vi "AP Quiz From File.vi"(8 "Error In":errorcluster, 11 "file path (dialog if empty)":path=path "C:/Users/husmith/Documents/GitHub/Action Pack/Quiz/QuizSetupSpreadsheet_Test.txt") -> (0 "Error Out":errorcluster, 1 "Raw Data":string[][](array[string]), 2 "Question Array Out":T1[](array[typedef]))   [LabVIEW 2012]
uses:
  Controls/Quiz Info.ctl
  Controls/Quiz Solution.ctl
  <vilib>/Utility/file.llb/Read From Spreadsheet File (string).vi
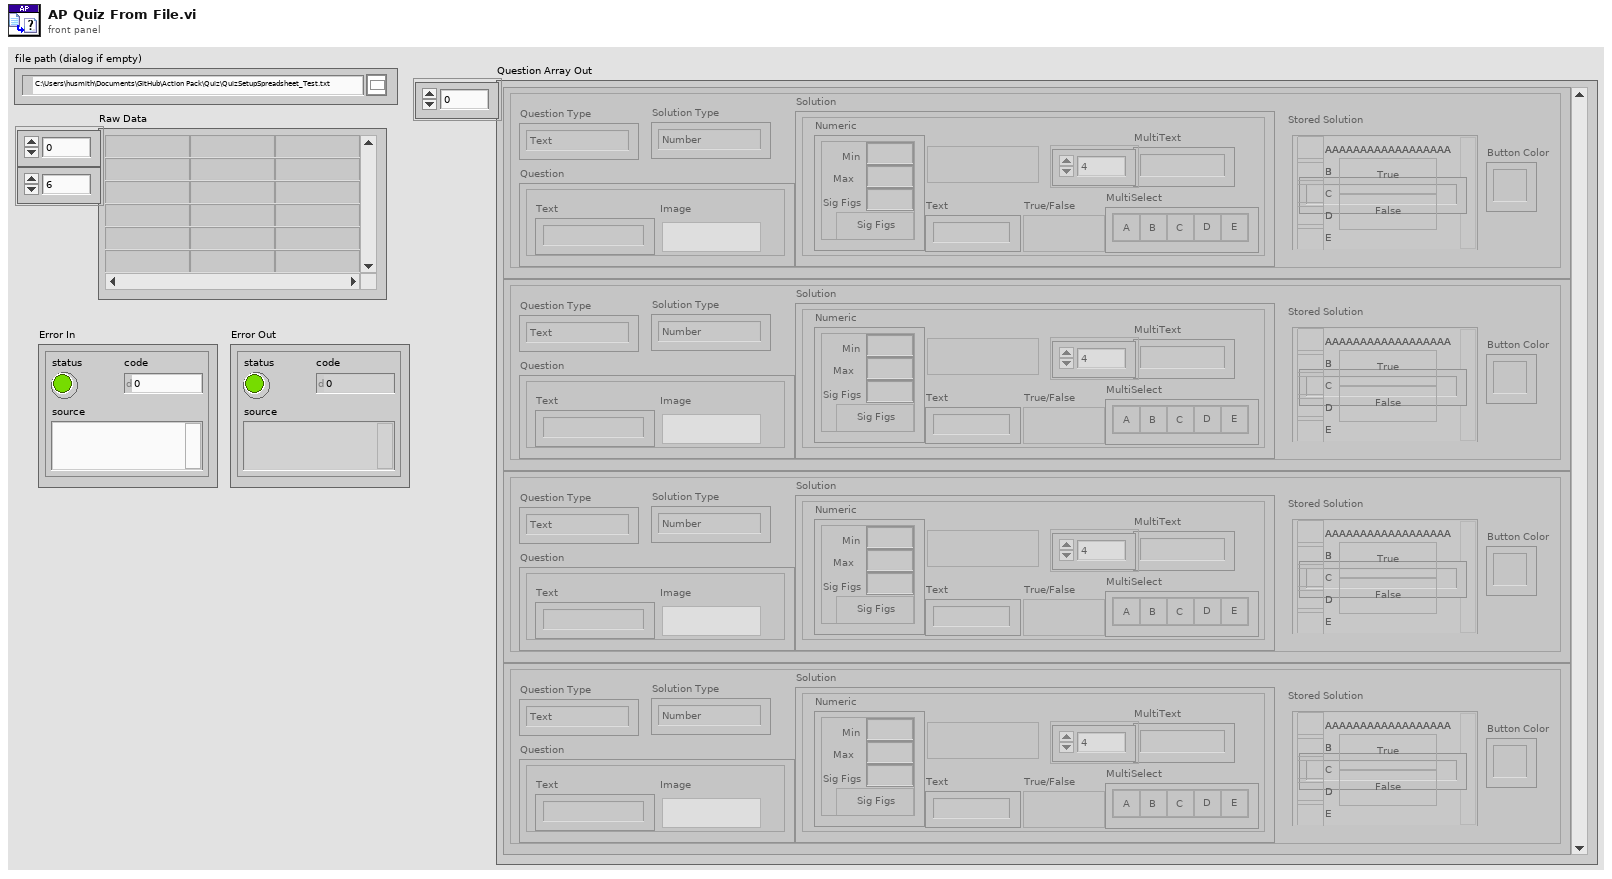
[diagram p1: front panel]
types:
  T1 = typedef "Quiz Info.ctl" = cluster{"Question Type":enum16{"Text", "Image", "Text&Image"}, "Solution Type":enum16{"Number", "Text", "MultiChoice", "Radio", "T/F", "Paragraph"}, "Question":cluster{"Text":string, "Image":picture}, "Solution":cluster{"Numeric":cluster{"Min":dbl, "Max":dbl, "Sig Figs":i32, "Sig Figs?":bool}, "Text":string, "True/False":bool, "MultiSelect":cluster{"A":bool, "B":bool, "C":bool, "D":bool, "E":bool}, "MultiText":string[], "Text Case Match":bool}, "Stored Solution":T2, "Button Color":u32}
  T2 = typedef "Quiz Solution.ctl" = cluster{"Numeric":dbl, "Text":string, "Multi":cluster{"A":bool, "B":bool, "C":bool, "D":bool, "E":bool}, "Radio":enum32{"No Selection", "A", "B", "C", "D", "E"}, "True/False":enum32{"No Selection", "True", "False"}, "Short Answer":string}
  T3 = enum16{"Number", "Text", "MultiChoice", "Radio", "T/F", "Paragraph"}
  T4 = typedef "imagedata.ctl" = cluster{"image type":i32, "image depth":i32, "image":u8[], "mask":u8[], "colors":u32[], "Rectangle":cluster{"left":i16, "top":i16, "right":i16, "bottom":i16}}
  T5 = cluster{"A":bool, "B":bool, "C":bool, "D":bool, "E":bool}
  T6 = cluster{"MultiSelect[0]":bool, "MultiSelect[1]":bool, "MultiSelect[2]":bool, "MultiSelect[3]":bool, "MultiSelect[4]":bool}
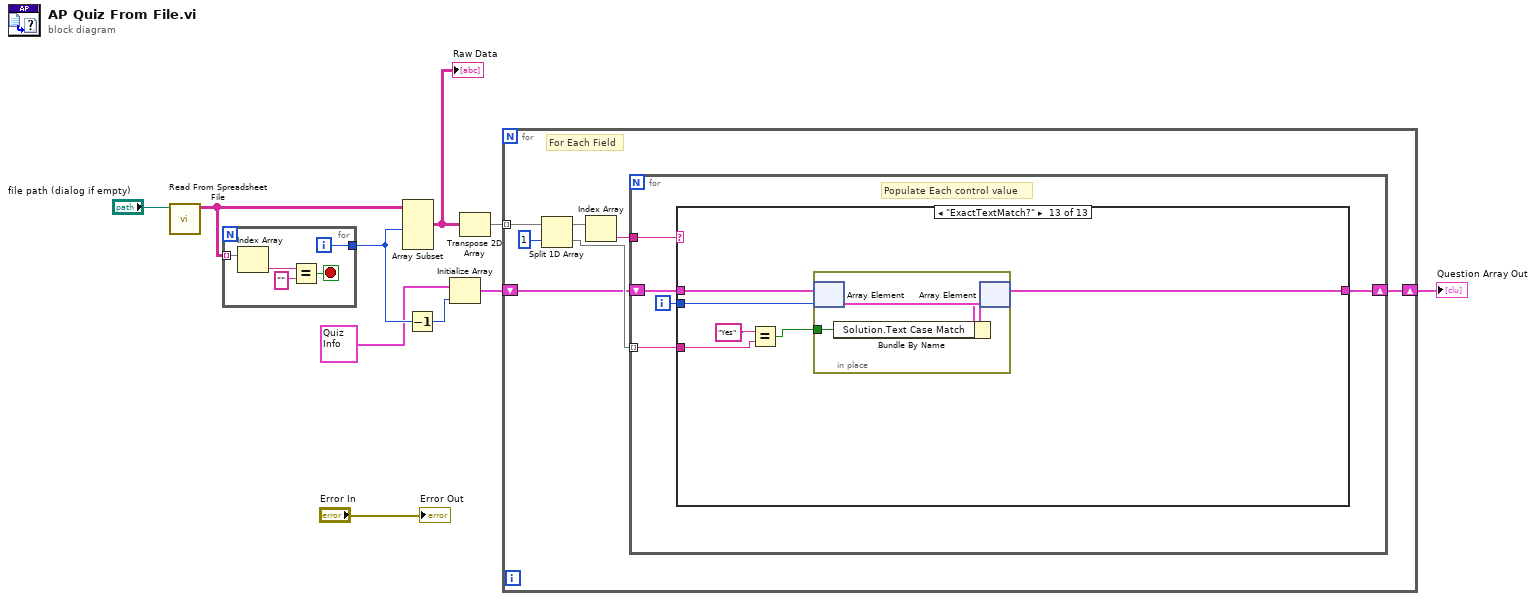
[diagram p0: block diagram]
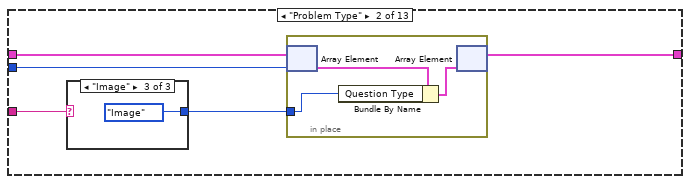
[diagram p3: hidden frame]
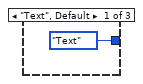
[diagram p4: hidden frame]
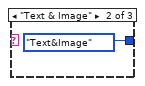
[diagram p5: hidden frame]
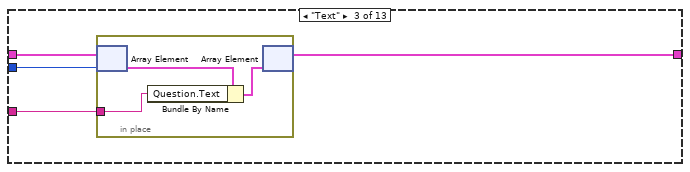
[diagram p6: hidden frame]
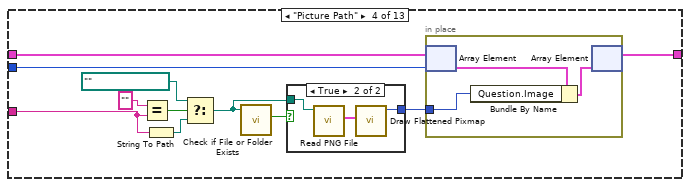
[diagram p7: hidden frame]
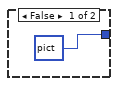
[diagram p8: hidden frame]
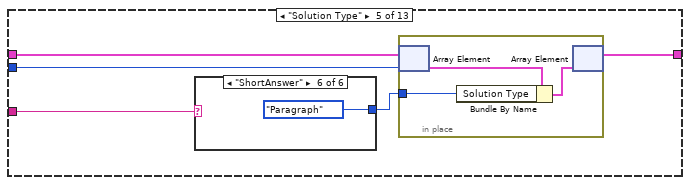
[diagram p9: hidden frame]
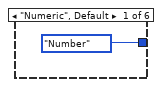
[diagram p10: hidden frame]
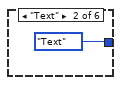
[diagram p11: hidden frame]
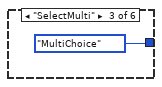
[diagram p12: hidden frame]
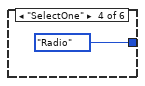
[diagram p13: hidden frame]
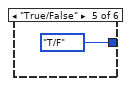
[diagram p14: hidden frame]
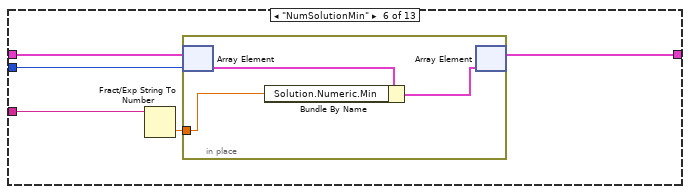
[diagram p15: hidden frame]
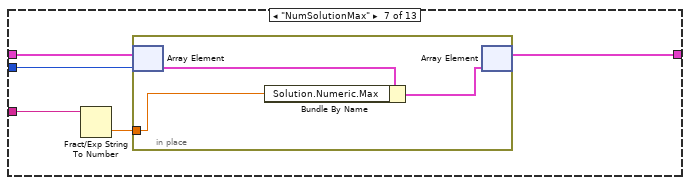
[diagram p16: hidden frame]
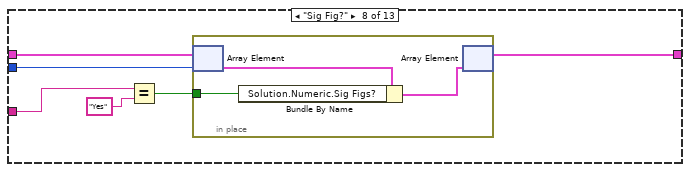
[diagram p17: hidden frame]
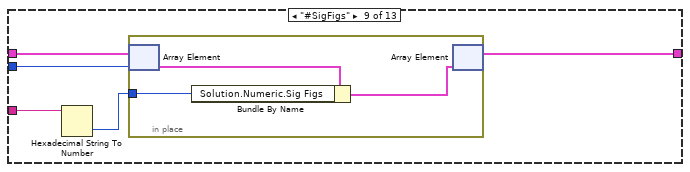
[diagram p18: hidden frame]
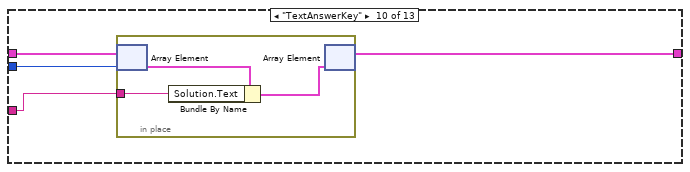
[diagram p19: hidden frame]
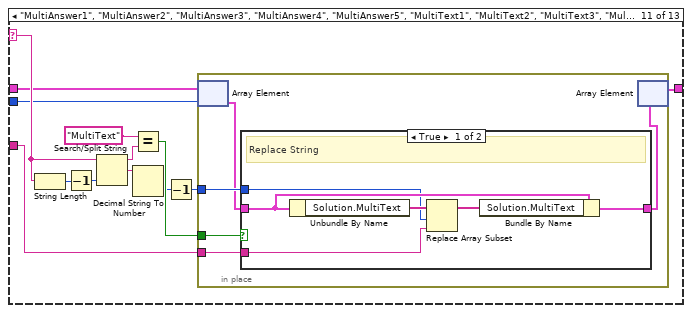
[diagram p20: hidden frame]
diagram:
  n1 = call-poly <vilib>:"Read From Spreadsheet File.vi"("file path (dialog if empty)"="file path (dialog if empty)") -> ("all rows"=w9:string[][])  [unwired: 6 in, 4 out]
  n2 = for {
    tunnel: [w14] -> w6
    tunnel: w9 -> [w13] mode=indexing
    i -> [w14]
    stop <- w11 stop-if-true
    n3 = Index Array(array=w13) -> (element=w12:string)  [unwired: 1 in]
    n4 = Equal?(x=w12, y="") -> (x = y?=w11:bool)
  }
  n5 = Array Subset(array=w9, length (row)=w6) -> (w5:string[][])  [unwired: 3 in]
  "Raw Data" <- w5
  n6 = Decrement(x=w6) -> (x-1=w7:i32)
  n7 = Initialize Array(T1 {"Question Type"=enum."Text", "Solution Type"=enum."Number", "Question"={"Text"="", "Image"=bytes[0]}, "Solution"={"Numeric"={"Min"=0.0, "Max"=0.0, "Sig Figs"=0, "Sig Figs?"=FALSE}, "Text"="", "True/False"=FALSE, "MultiSelect"={"A"=FALSE, "B"=FALSE, "C"=FALSE, "D"=FALSE, "E"=FALSE}, "MultiText"=["", "", "", "", ""], "Text Case Match"=FALSE}, "Stored Solution"={"Numeric"=0.0, "Text"="", "Multi"={"A"=FALSE, "B"=FALSE, "C"=FALSE, "D"=FALSE, "E"=FALSE}, "Radio"=enum."No Selection", "True/False"=enum."No Selection", "Short Answer"=""}, "Button Color"=14869218} ("Quiz Info"), w7) -> (w8:T1[])
  n8 = Transpose 2D Array(2D array=w5) -> (transposed array=w10:string[][])
  n9 = for {
    tunnel: w10 -> [w22] mode=indexing
    shift-right: [w16] -> w1
    shift-left: w8 -> [w18]
    # "For Each Field"
    n10 = Split 1D Array(array=w22, index=1) -> (first subarray=w19:string[], second subarray=w20:string[])
    n11 = Index Array(array=w19) -> (element=w17:string)  [unwired: 1 in]
    n12 = for {
      tunnel: w20 -> [w27] mode=indexing
      tunnel: w17 -> [w26]
      shift-right: [w24] -> w16
      shift-left: w18 -> [w25]
      i -> [w23]
      # "Populate Each control value"
      n13 = case shown="\"ExactTextMatch?\"" w26 {
        selector: w26 -> [_ _ _ _ _ _ _ _ _ _ w126 _ _]
        tunnel: w27 -> [_ w33 w40 w52 w67 w83 w91 w97 w105 w112 w120 w155 w164]
        tunnel: w25 -> [w28 w32 w43 w56 w69 w81 w89 w99 w107 w114 w125 w157 w167]
        tunnel: [w28 w31 w42 w57 w68 w79 w87 w98 w106 w113 w119 w158 w166] -> w24
        tunnel: w23 -> [_ w29 w41 w54 w65 w82 w90 w100 w108 w115 w124 w156 w162]
        frame "NULL", Default {
        }
        frame "Problem Type" {
          n14 = case shown="\"Image\"" w33 {
            tunnel: [enum16{"Text", "Image", "Text&Image"}."Text" ("Question Type") enum16{"Text", "Image", "Text&Image"}."Text&Image" ("Question Type") enum16{"Text", "Image", "Text&Image"}."Image" ("Question Type")] -> w30
            frame "Text", Default {
            }
            frame "Text & Image" {
            }
            frame "Image" {
            }
          }
          n15 = in-place {
            in-place-border: w30 -> [w34]
            n16 = in-place-array #1(w32, w29) -> (w36:T1)
            n17 = Bundle By Name(cluster=w36, "Question Type"=w34) -> (w35:T1)
            n18 = in-place-array #1(w35) -> (w31:T1[])  [unwired: 1 out]
          }
        }
        frame "Text" {
          n19 = in-place {
            in-place-border: w40 -> [w44]
            n20 = in-place-array #2(w43, w41) -> (w46:T1)
            n21 = Bundle By Name(cluster=w46, "Question.Text"=w44) -> (w45:T1)
            n22 = in-place-array #2(w45) -> (w42:T1[])  [unwired: 1 out]
          }
        }
        frame "Picture Path" {
          n23 = Equal?(x="", y=w52) -> (x = y?=w50:bool)
          n24 = String To Path(string=w52) -> (path=w49:path)
          n25 = Select(t=path "", s=w50, f=w49) -> (s? t:f=w48:path)
          n26 = call <vilib>:"Check if File or Folder Exists.vi"("path"=w48) -> ("file or folder exists?"=w53:bool)  [unwired: 8 in, 2 out]
          n27 = case shown="True" w53 {
            tunnel: [picture data[5B] ("new picture") w60] -> w55
            tunnel: w48 -> [_ w59]
            frame False {
            }
            frame True {
              n28 = call <vilib>:"Read PNG File.vi"("path to PNG file"=w59) -> ("image data"=w61:T4)  [unwired: 8 in, 2 out]
              n29 = call <vilib>:"Draw Flattened Pixmap.vi"("image data"=w61) -> ("new picture"=w60:picture)  [unwired: 8 in]
            }
          }
          n30 = in-place {
            in-place-border: w55 -> [w62]
            n31 = in-place-array #3(w56, w54) -> (w64:T1)
            n32 = Bundle By Name(cluster=w64, "Question.Image"=w62) -> (w63:T1)
            n33 = in-place-array #3(w63) -> (w57:T1[])  [unwired: 1 out]
          }
        }
        frame "Solution Type" {
          n34 = case shown="\"ShortAnswer\"" w67 {
            tunnel: [T3."Number" ("Solution Type") T3."Text" ("Solution Type") T3."MultiChoice" ("Solution Type") T3."Radio" ("Solution Type") T3."T/F" ("Solution Type") T3."Paragraph" ("Solution Type")] -> w66
            frame "Numeric", Default {
            }
            frame "Text" {
            }
            frame "SelectMulti" {
            }
            frame "SelectOne" {
            }
            frame "True/False" {
            }
            frame "ShortAnswer" {
            }
          }
          n35 = in-place {
            in-place-border: w66 -> [w76]
            n36 = in-place-array #4(w69, w65) -> (w78:T1)
            n37 = Bundle By Name(cluster=w78, "Solution Type"=w76) -> (w77:T1)
            n38 = in-place-array #4(w77) -> (w68:T1[])  [unwired: 1 out]
          }
        }
        frame "NumSolutionMin" {
          n39 = Fract/Exp String To Number(string=w83) -> (number=w80:dbl)  [unwired: 3 in, 1 out]
          n40 = in-place {
            in-place-border: w80 -> [w84]
            n41 = in-place-array #5(w81, w82) -> (w86:T1)
            n42 = Bundle By Name(cluster=w86, "Solution.Numeric.Min"=w84) -> (w85:T1)
            n43 = in-place-array #5(w85) -> (w79:T1[])  [unwired: 1 out]
          }
        }
        frame "NumSolutionMax" {
          n44 = Fract/Exp String To Number(string=w91) -> (number=w88:dbl)  [unwired: 3 in, 1 out]
          n45 = in-place {
            in-place-border: w88 -> [w92]
            n46 = in-place-array #6(w89, w90) -> (w94:T1)
            n47 = Bundle By Name(cluster=w94, "Solution.Numeric.Max"=w92) -> (w93:T1)
            n48 = in-place-array #6(w93) -> (w87:T1[])  [unwired: 1 out]
          }
        }
        frame "Sig Fig?" {
          n49 = Equal?(x=w97, y="Yes") -> (x = y?=w95:bool)
          n50 = in-place {
            in-place-border: w95 -> [w101]
            n51 = in-place-array #7(w99, w100) -> (w103:T1)
            n52 = Bundle By Name(cluster=w103, "Solution.Numeric.Sig Figs?"=w101) -> (w102:T1)
            n53 = in-place-array #7(w102) -> (w98:T1[])  [unwired: 1 out]
          }
        }
        frame "#SigFigs" {
          n54 = Hexadecimal String To Number(string=w105) -> (number=w104:u32)  [unwired: 2 in, 1 out]
          n55 = in-place {
            in-place-border: w104 -> [w109]
            n56 = in-place-array #8(w107, w108) -> (w111:T1)
            n57 = Bundle By Name(cluster=w111, "Solution.Numeric.Sig Figs"=w109) -> (w110:T1)
            n58 = in-place-array #8(w110) -> (w106:T1[])  [unwired: 1 out]
          }
        }
        frame "TextAnswerKey" {
          n59 = in-place {
            in-place-border: w112 -> [w116]
            n60 = in-place-array #9(w114, w115) -> (w118:T1)
            n61 = Bundle By Name(cluster=w118, "Solution.Text"=w116) -> (w117:T1)
            n62 = in-place-array #9(w117) -> (w113:T1[])  [unwired: 1 out]
          }
        }
        frame "MultiAnswer1", "MultiAnswer2", "MultiAnswer3", "MultiAnswer4", "MultiAnswer5", "MultiText1", "MultiText2", "MultiText3", "MultiText4", "MultiText5" {
          n63 = String Length(string=w126) -> (length=w130:i32)
          n64 = Decrement(x=w130) -> (x-1=w129:i32)
          n65 = Search/Split String(string=w126, offset (0)=w129) -> (substring before match=w128:string, match + rest of string=w131:string)  [unwired: 1 in, 1 out]
          n66 = Equal?(x="MultiText" ("String"), y=w128) -> (x = y?=w123:bool)
          n67 = Decimal String To Number(string=w131) -> (number=w122:i32)  [unwired: 2 in, 1 out]
          n68 = Decrement(x=w122) -> (x-1=w121:i32)
          n69 = in-place {
            in-place-border: w123 -> [w136]
            in-place-border: w121 -> [w135]
            in-place-border: w120 -> [w134]
            n70 = in-place-array #10(w125, w124) -> (w133:T1)
            n71 = case shown="True" w136 {
              tunnel: w133 -> [w141 w152]
              tunnel: [w139 w151] -> w132
              tunnel: w135 -> [w138 w143]
              tunnel: w134 -> [w137 w149]
              frame True {
                # "Replace String"
                n72 = Unbundle By Name(w141) -> ("Solution.MultiText"=w142:string[])
                n73 = Replace Array Subset(array=w142, new element=w137, index=w138) -> (w140:string[])
                n74 = Bundle By Name(cluster=w141, "Solution.MultiText"=w140) -> (w139:T1)
              }
              frame False {
                # "Replace Bool"
                n75 = Unbundle By Name(w152) -> ("Solution.MultiSelect"=w148:T5)
                n76 = Equal?(x=w149, y="TRUE") -> (x = y?=w144:bool)
                n77 = Cluster To Array(cluster=w148) -> (array=w147:bool[])
                n78 = Replace Array Subset(array=w147, new element=w144, index=w143) -> (w146:bool[])
                n79 = Array To Cluster(array=w146) -> (cluster=w145:T6)
                n80 = Bundle By Name(cluster=w152, "Solution.MultiSelect"=w145) -> (w151:T1)
              }
            }
            n81 = in-place-array #10(w132) -> (w119:T1[])  [unwired: 1 out]
          }
        }
        frame "T/F_Answer" {
          n82 = Equal?(x="TRUE" ("y"), y=w155) -> (x = y?=w153:bool)
          n83 = in-place {
            in-place-border: w153 -> [w159]
            n84 = in-place-array #11(w157, w156) -> (w161:T1)
            n85 = Bundle By Name(cluster=w161, "Solution.True/False"=w159) -> (w160:T1)
            n86 = in-place-array #11(w160) -> (w158:T1[])  [unwired: 1 out]
          }
        }
        frame "ExactTextMatch?" {
          n87 = Equal?(x="Yes" ("y"), y=w164) -> (x = y?=w163:bool)
          n88 = in-place {
            in-place-border: w163 -> [w168]
            n89 = in-place-array #12(w167, w162) -> (w170:T1)
            n90 = Bundle By Name(cluster=w170, "Solution.Text Case Match"=w168) -> (w169:T1)
            n91 = in-place-array #12(w169) -> (w166:T1[])  [unwired: 1 out]
          }
        }
      }
    }
  }
  "Question Array Out" <- w1
  "Error Out" <- "Error In"
